vi "Vision Tracking Values.vi"() -> (4 "Center":dbl, 5 "Distance (ft)":dbl)   [LabVIEW 2015]
uses:
  Vision/Vision Global.vi
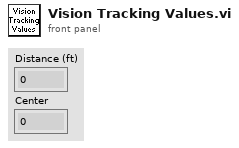
[diagram p1: front panel]
types:
  T1 = cluster{"Distance (ft)":dbl, "Center":cluster{dbl, dbl}, "Normalized Rect":cluster{"Numeric":dbl, "Numeric 2":dbl, "Numeric 3":dbl, "Numeric 5":dbl}}[]
  T2 = cluster{"Distance (ft)":dbl, "Center":cluster{dbl, dbl}, "Normalized Rect":cluster{"Numeric":dbl, "Numeric 2":dbl, "Numeric 3":dbl, "Numeric 5":dbl}}
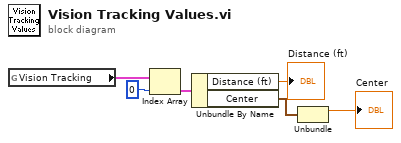
[diagram p0: block diagram]
diagram:
  n1 = global read "Vision Global.vi" "Vision Tracking"() -> (w4:T1)
  n2 = Index Array(array=w4, index=0) -> (element=w5:T2)
  n3 = Unbundle By Name(w5) -> ("Distance (ft)"=→"Distance (ft)":dbl, "Center"=w2:cluster{dbl, dbl})
  n4 = Unbundle(w2) -> (→"Center":dbl)  [unwired: 1 out]
